vi "Create Register.vi"() -> ()   [LabVIEW 2011]
uses:
  <vilib>/registry/registry.llb/Registry RtKey.ctl
  <vilib>/registry/registry.llb/Write Registry Value Simple STR.vi
  <vilib>/registry/registry.llb/Write Registry Value Simple U32.vi
panel:
  in  "Info":T1
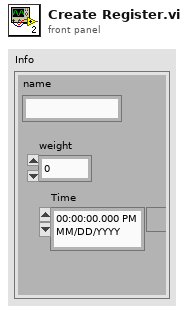
[diagram p1: front panel]
types:
  T1 = cluster{"name":string, "weight":u64, "Time":timestamp}
  T2 = typedef "Registry RtKey.ctl" = enum32{"HKEY_CLASSES_ROOT", "HKEY_CURRENT_USER", "HKEY_LOCAL_MACHINE", "HKEY_USERS", "HKEY_PERFORMANCE_DATA", "HKEY_CURRENT_CONFIG", "HKEY_DYN_DATA"}
  T3 = typedef "Registry refnum.ctl" = refnum<k1>
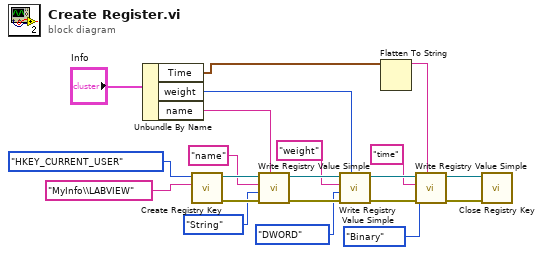
[diagram p0: block diagram]
diagram:
  n1 = Unbundle By Name("Info") -> ("Time"=w2:timestamp, "weight"=w3:u64, "name"=w4:string)
  n2 = call <vilib>:"Create Registry Key.vi"("subkey"="MyInfo\\LABVIEW", "root key (HKEY_LOCAL_MACHINE)"=Registry_RtKey."HKEY_CURRENT_USER") -> ("error out"=w20:errorcluster, "refnum out"=w21:T3)  [unwired: 7 in, 1 out]
  n3 = call-poly <vilib>:"Write Registry Value Simple.vi"("String/Binary data"=w4, "error in (no error)"=w20, "simple data type"=enum16{"String", "Binary", "DWORD"}."String", "value"="name", "refnum"=w21) -> ("error out"=w18:errorcluster, "refnum out"=w19:T3)  [unwired: 3 in]
  n4 = call-poly <vilib>:"Write Registry Value Simple.vi"("DWORD data"=w3, "error in (no error)"=w18, "simple data type"=enum16{"String", "Binary", "DWORD"}."DWORD", "value"="weight", "refnum"=w19) -> ("error out"=w17:errorcluster, "refnum out"=w16:T3)  [unwired: 3 in]
  n5 = Flatten To String(anything=w2) -> (data string=w1:string)  [unwired: 3 in, 2 out]
  n6 = call-poly <vilib>:"Write Registry Value Simple.vi"("String/Binary data"=w1, "error in (no error)"=w17, "simple data type"=enum16{"String", "Binary", "DWORD"}."Binary", "value"="time", "refnum"=w16) -> ("error out"=w14:errorcluster, "refnum out"=w15:T3)  [unwired: 3 in]
  n7 = call <vilib>:"Close Registry Key.vi"("error in (no error)"=w14, "refnum"=w15) -> ()  [unwired: 5 in, 1 out]
